vi "write control value - polymorphic.vi"   [LabVIEW 2024, in "controls manager.lvlib"]
uses:
  controls manager.lvlib
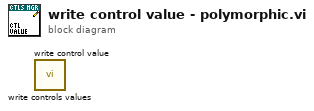
[diagram p0: block diagram]
diagram:
  n1 = call "write controls values.vi"() -> ()  [unwired: 11 in, 1 out]
  n2 = call "write control value.vi"() -> ()  [unwired: 11 in, 1 out]
